vi "Re-sample Waveform.vi"(8 "Error":errorcluster, 9 "Waveform":T1, 11 "WavBuf":refnum<class "WavBuf.lvclass">) -> (0 "Error Out":errorcluster, 1 "Waveform Out":T1, 3 "WavBuf Out":refnum<class "WavBuf.lvclass">)   [LabVIEW 2024, in "WavBuf.lvclass"]
uses:
  WavBuf.lvclass
  Universal Controls/Waveform_Data.ctl
  WavBuf.lvclass/WavBuf.ctl
  Support/Measure_Decimate Dbl Array.vi
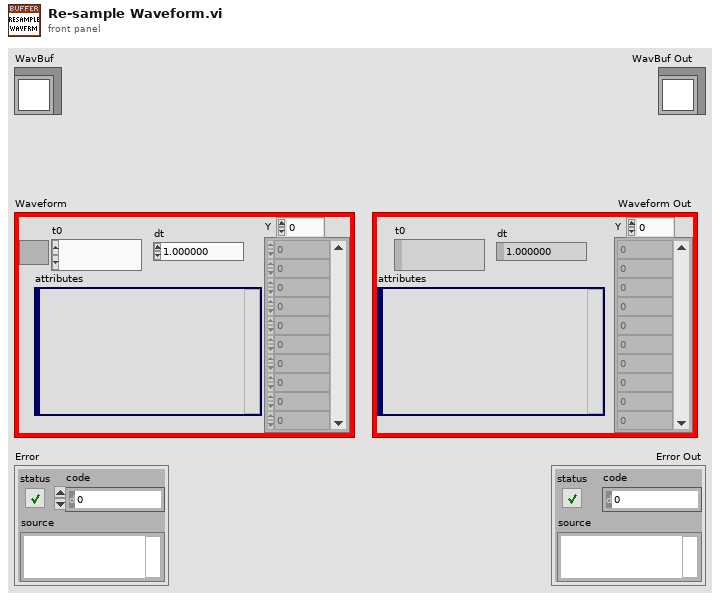
[diagram p1: front panel]
types:
  T1 = typedef "Waveform_Data.ctl" = waveform(dbl)
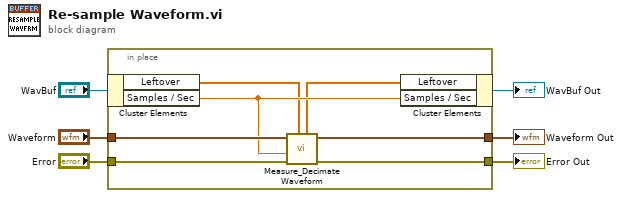
[diagram p0: block diagram]
diagram:
  n1 = in-place {
    in-place-border: [w9] -> w6
    in-place-border: [w13] -> w5
    in-place-border: "Waveform" -> [w12]
    in-place-border: "Error" -> [w11]
    n2 = in-place-cluster #1("WavBuf") -> ("Leftover"=w8:dbl[], "Samples / Sec"=w10:dbl)
    n3 = call "Measure_Decimate Waveform.vi"("Leftover last"=w8, "Error"=w11, "Target Sample Rate"=w10, "Waveform To Decimate"=w12) -> ("Error Out"=w13:errorcluster, "Waveform Out"=w9:T1, "Leftover Out"=w7:dbl[])  [unwired: 5 in]
    n4 = in-place-cluster #1("Leftover"=w7, "Samples / Sec"=w10) -> (→"WavBuf Out":refnum<class "WavBuf.lvclass">)
  }
  "Waveform Out" <- w6
  "Error Out" <- w5
